vi "SeqMgr.For Statement, Find Next.vi"(9 "Arguements":string[](array[string]), 10 "Next Step":i32, 11 "Sequence":string[][](array[string])) -> (0 "error out":errorcluster, 2 "Next Step":i32, 3 "End":bool)   [LabVIEW 2024, in "EQMF.lvlib" / "SeqMgr.lvlib"]
uses:
  SeqMgr.lvlib
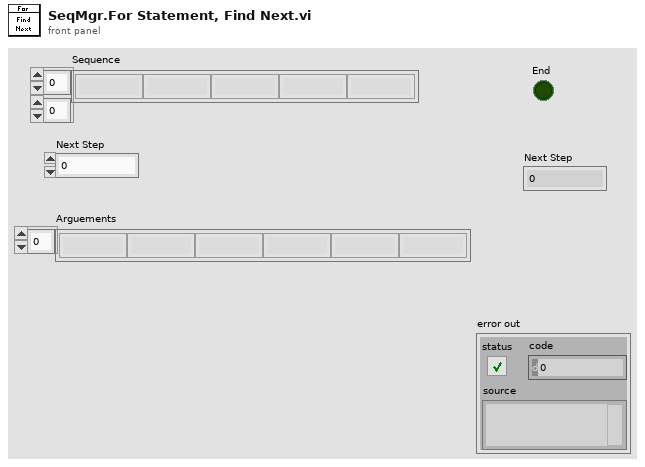
[diagram p1: front panel]
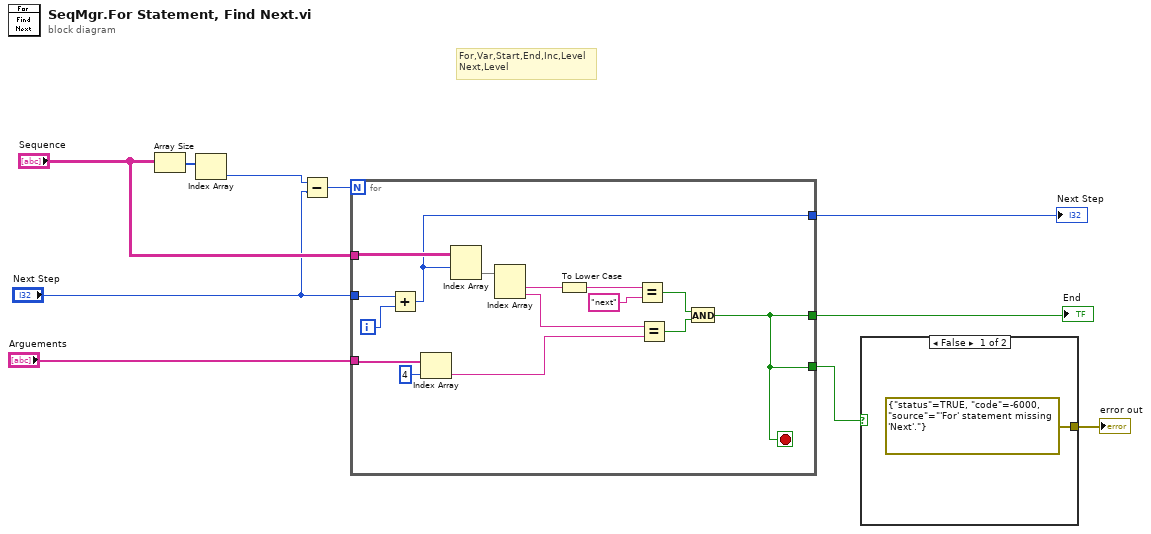
[diagram p0: block diagram]
diagram:
  # "For,Var,Start,End,Inc,Level\nNext,Level"
  n1 = Array Size(array="Sequence") -> (size(s)=w6:i32[])
  n2 = Index Array(array=w6) -> (element=w1:i32)  [unwired: 1 in]
  n3 = Subtract(x=w1, y="Next Step") -> (x-y=w5:i32)
  n4 = for {
    N: w5 -> [_]
    tunnel: "Next Step" -> [w25]
    tunnel: "Sequence" -> [w23]
    tunnel: "Arguements" -> [w20]
    tunnel: [w14] -> w8
    tunnel: [w13] -> w4
    tunnel: [w13] -> w3
    i -> [w24]
    stop <- w13 stop-if-true
    n5 = Add(x=w25, y=w24) -> (x+y=w14:i32)
    n6 = Index Array(array=w20, index=4) -> (element=w15:string)
    n7 = Index Array(array=w23, index (row)=w14) -> (element=w22:string[])  [unwired: 1 in]
    n8 = Index Array(array=w22) -> (element #1=w12:string, element #2=w16:string)  [unwired: 2 in]
    n9 = To Lower Case(string=w12) -> (all lower case string=w11:string)
    n10 = Equal?(x=w11, y="next") -> (x = y?=w18:bool)
    n11 = Equal?(x=w16, y=w15) -> (x = y?=w17:bool)
    n12 = And(x=w18, y=w17) -> (x .and. y?=w13:bool)
  }
  "End" <- w4
  "Next Step" <- w8
  n13 = case shown="False" w3 {
    tunnel: [errorcluster {"status"=TRUE, "code"=-6000, "source"="'For' statement missing 'Next'."} ("error constant") _] -> w2
    frame False {
    }
    frame True {
    }
  }
  "error out" <- w2
